vi "Build Tree.vi"(8 "error in (no error)":errorcluster, 9 "No Project Text Reference":refnum<vi>, 10 "Tree Reference In":refnum<vi>, 11 "CS++MessageMakerMain in":refnum<class "CS++MessageMakerMain.lvclass">) -> (0 "error out":errorcluster, 2 "Tree Reference Out":refnum<vi>, 3 "CS++MessageMakerMain out":refnum<class "CS++MessageMakerMain.lvclass">)   [LabVIEW 2014, in "CS++MessageMakerMain.lvlib" / "CS++MessageMakerMain.lvclass"]
doc: "Updates the Tree on the Front Panel."
uses:
  CS++MessageMakerMain.lvclass
  CS++MessageMakerMain.lvclass/CS++MessageMakerMain.ctl
  CSPP_Actor/CS++Actor.lvclass/CS++Actor.ctl
  CSPP_Method/CS++Method.lvclass/CS++Method.ctl
  CSPP_Message/CS++Message.lvclass/CS++Message.ctl
  CSPP_Actor/CS++Actor.lvclass
  CSPP_Method/CS++Method.lvclass
  CSPP_Message/CS++Message.lvclass
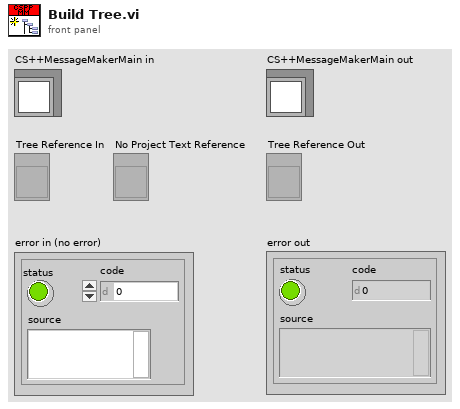
[diagram p1: front panel]
types:
  T1 = cluster{"Left Cell String":string, "Child Text":string[], "Child Tag":string, "Item Indent":i32, "Child Only?":bool, "Glyph Index":i32}
  T2 = cluster{"Left Cell String":string, "Child Text":string[], "Child Tag":string, "Item Indent":i32, "Child Only?":bool, "Glyph Index":i32}[]
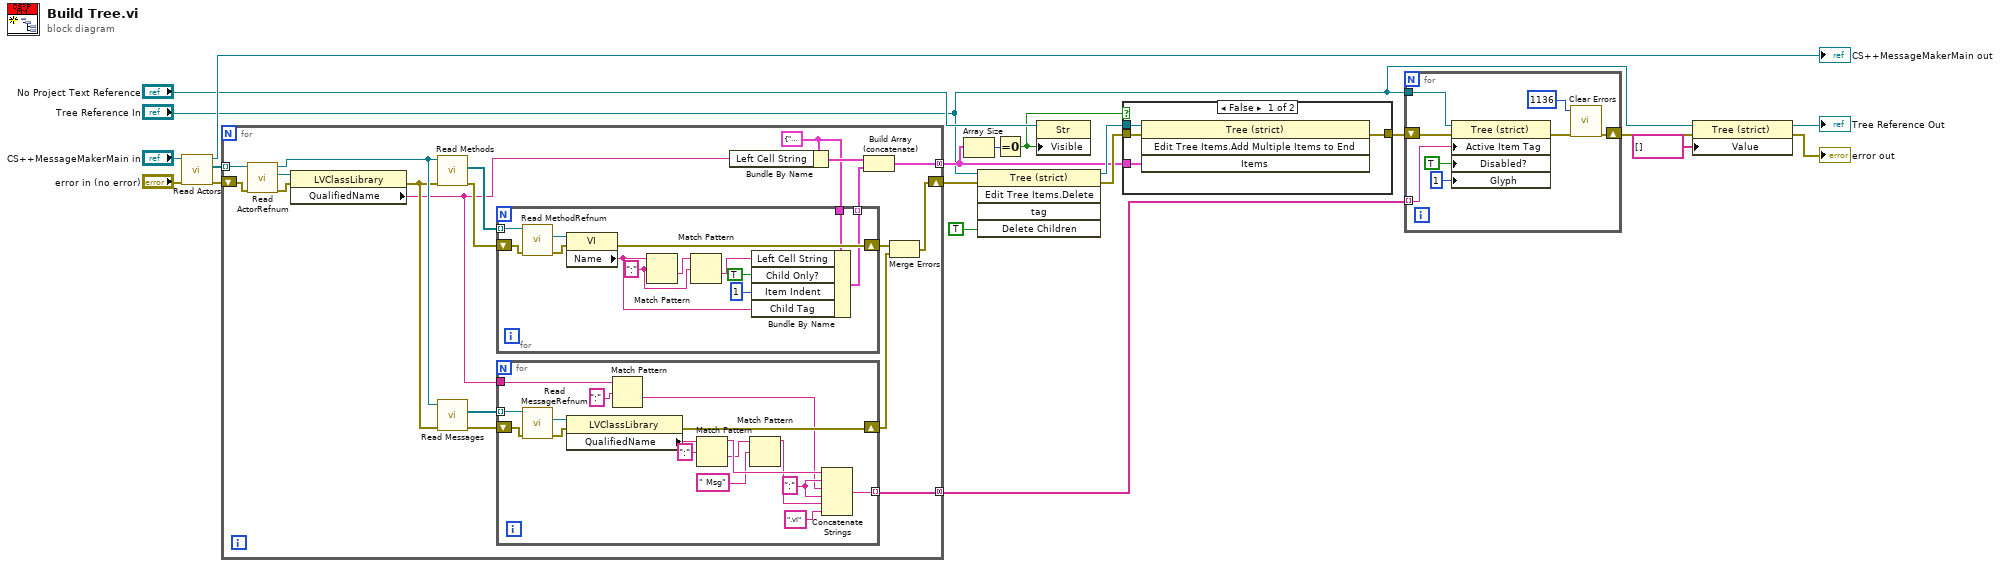
[diagram p0: block diagram]
diagram:
  n1 = call "Read Actors.vi"("error in (no error)"="error in (no error)", "CS++MessageMakerMain in"="CS++MessageMakerMain in") -> ("error out"=w19:errorcluster, "Actors"=w20:refnum<class "CS++Actor.lvclass">[], "CS++MessageMakerMain out"=→"CS++MessageMakerMain out":refnum<class "CS++MessageMakerMain.lvclass">)  [unwired: 7 in]
  n2 = for {
    tunnel: w20 -> [w37] mode=indexing
    shift-right: [w21] -> w17
    shift-left: w19 -> [w38]
    tunnel: [w31] -> w15 mode=concatenating
    tunnel: [w24] -> w11 mode=concatenating
    w32 = T1 {"Left Cell String"="", "Child Text"=[], "Child Tag"="", "Item Indent"=0, "Child Only?"=FALSE, "Glyph Index"=0} ("Item")
    n3 = call "Read ActorRefnum.vi"("error in (no error)"=w38, "CS++Actor in"=w37) -> ("error out"=w35:errorcluster, "ActorRefnum"=w36:refnum<vi>, "CS++Actor out"=w29:refnum<class "CS++Actor.lvclass">)  [unwired: 7 in]
    n4 = property class="LVClassLibrary"(reference=w36, error in=w35) -> (error out=w28:errorcluster, "QualifiedName"=w25:string)  [unwired: 1 out]
    n5 = call "Read Methods.vi"("error in (no error)"=w28, "CS++Actor in"=w29) -> ("error out"=w34:errorcluster, "Methods"=w33:refnum<class "CS++Method.lvclass">[])  [unwired: 7 in, 1 out]
    n6 = call "Read Messages.vi"("error in (no error)"=w28, "CS++Actor in"=w29) -> ("error out"=w26:errorcluster, "Messages"=w27:refnum<class "CS++Message.lvclass">[])  [unwired: 7 in, 1 out]
    n7 = for {
      shift-right: [w65] -> w23
      shift-left: w34 -> [w69]
      tunnel: w33 -> [w68] mode=indexing
      tunnel: w32 -> [w64]
      tunnel: [w61] -> w30 mode=indexing
      w59 = ":"
      n8 = call "Read MethodRefnum.vi"("error in (no error)"=w69, "CS++Methods in"=w68) -> ("error out"=w66:errorcluster, "MethodRefnum"=w67:refnum<vi>)  [unwired: 7 in, 1 out]
      n9 = property class="VI"(reference=w67, error in=w66) -> (error out=w65:errorcluster, "Name"=w57:string)  [unwired: 1 out]
      n10 = Match Pattern(string=w57, regular expression=w59) -> (after substring=w60:string)  [unwired: 1 in, 3 out]
      n11 = Match Pattern(string=w60, regular expression=w59) -> (after substring=w58:string)  [unwired: 1 in, 3 out]
      n12 = Bundle By Name(cluster=w64, "Left Cell String"=w58, "Child Only?"=TRUE, "Item Indent"=1, "Child Tag"=w57) -> (w61:T1)
    }
    n13 = for {
      tunnel: w27 -> [w56] mode=indexing
      shift-right: [w52] -> w22
      shift-left: w26 -> [w55]
      tunnel: w25 -> [w46]
      tunnel: [w48] -> w24 mode=indexing
      w41 = ":" ("string")
      n14 = call "Read MessageRefnum.vi"("error in (no error)"=w55, "CS++Message in"=w56) -> ("error out"=w53:errorcluster, "MessageRefnum"=w54:refnum<vi>)  [unwired: 7 in, 1 out]
      n15 = property class="LVClassLibrary"(reference=w54, error in=w53) -> (error out=w52:errorcluster, "QualifiedName"=w50:string)  [unwired: 1 out]
      n16 = Match Pattern(string=w46, regular expression=":") -> (after substring=w40:string)  [unwired: 1 in, 3 out]
      n17 = Match Pattern(string=w50, regular expression=":") -> (before substring=w49:string, after substring=w43:string)  [unwired: 1 in, 2 out]
      n18 = Match Pattern(string=w43, regular expression=" Msg") -> (before substring=w42:string)  [unwired: 1 in, 3 out]
      n19 = Concatenate Strings(w49, w41, w40, w41, w42, ".vi" ("string")) -> (w48:string)
    }
    n20 = Bundle By Name(cluster=w32, "Left Cell String"=w25) -> (w39:T1)
    n21 = Build Array (concatenate)(w39, w30) -> (w31:T2)
    n22 = Merge Errors(w23, w22) -> (w21:errorcluster)
  }
  n23 = Array Size(array=w15) -> (size(s)=w14:i32)
  n24 = invoke class="Tree (strict)" method="Edit Tree Items.Delete"(reference="Tree Reference In", error in=w17, "Delete Children"=TRUE ("Delete Children?")) -> (reference out=w18:refnum<vi>, error out=w16:errorcluster)  [unwired: 2 in, 3 out]
  n25 = Equal To 0?(x=w14) -> (x = 0?=w3:bool)
  n26 = property on="Property Node" class="Str"(reference="No Project Text Reference", "Visible"=w3) -> ()  [unwired: 1 in, 2 out]
  n27 = case shown="False" w3 {
    tunnel: w18 -> [w73 _]
    tunnel: w16 -> [w72 w74]
    tunnel: w15 -> [w71 _]
    tunnel: [w70 w74] -> w12
    frame False {
      n28 = invoke on="Invoke Node" class="Tree (strict)" method="Edit Tree Items.Add Multiple Items to End"(reference=w73, error in=w72, "Items"=w71) -> (error out=w70:errorcluster)  [unwired: 1 in, 3 out]
    }
    frame True {
    }
  }
  n29 = for {
    shift-right: [w77] -> w6
    shift-left: w12 -> [w80]
    tunnel: w11 -> [w81] mode=indexing
    tunnel: "Tree Reference In" -> [w79]
    n30 = property class="Tree (strict)"(reference=w79, error in=w80, "Active Item Tag"=w81, "Disabled?"=TRUE ("Active Item:Disabled?"), "Glyph"=1 ("Active Item:Symbol Index")) -> (error out=w78:errorcluster)  [unwired: 1 out]
    n31 = call <vilib>:"Clear Errors.vi"("error in (no error)"=w78, "specific error code to clear (0: all)"=1136) -> ("error out"=w77:errorcluster)  [unwired: 4 in, 1 out]
  }
  n32 = property class="Tree (strict)"(reference="Tree Reference In", error in=w6, "Value"=string[] []) -> (reference out=→"Tree Reference Out":refnum<vi>, error out=→"error out":errorcluster)
